vi "GDSAPI_SetClassOptions.vi"(8 "error in (no error)":errorcluster, 9 "WireConfiguration":T1={"Edge thickness"=1, "Edge color"=5667411, "Center thickness"=1, "Center pattern"=enum."Solid", "CenterColor1"=9740924, "CenterColor2"=8694662, "Tunnels and terminals colors"=131187}, 10 "PatternIn":T3 items=["4x4x4", "5x6x5", "6x8x6"], 11 "ProjectIconType":T4=enum."BlueFull") -> (0 "error out":errorcluster, 1 "WireConfiguration-Before":T1={"Edge thickness"=1, "Edge color"=5667411, "Center thickness"=1, "Center pattern"=enum."Solid", "CenterColor1"=9740924, "CenterColor2"=8694662, "Tunnels and terminals colors"=131187}, 2 "Pattern-Before":T3 items=["4x4x4", "5x6x5", "6x8x6"], 3 "ProjectIcon-Before":T4=enum."BlueFull")   [LabVIEW 2012]
uses:
  <resource>/Framework/Providers/Open_GDS/API/GDSAPI_SubVIs/GDSAPI_ProjectIconType.ctl
  <resource>/Framework/Providers/Open_GDS/ClassProviders/Common/ScriptingFunctions/Scripting_ConnectorPanePatternType.ctl
  <resource>/Framework/Providers/Open_GDS/SubVIs/GOOP_WireConfigurationType.ctl
  <resource>/Framework/Providers/Open_GDS/SubVIs/GOOP_WirePattern.ctl
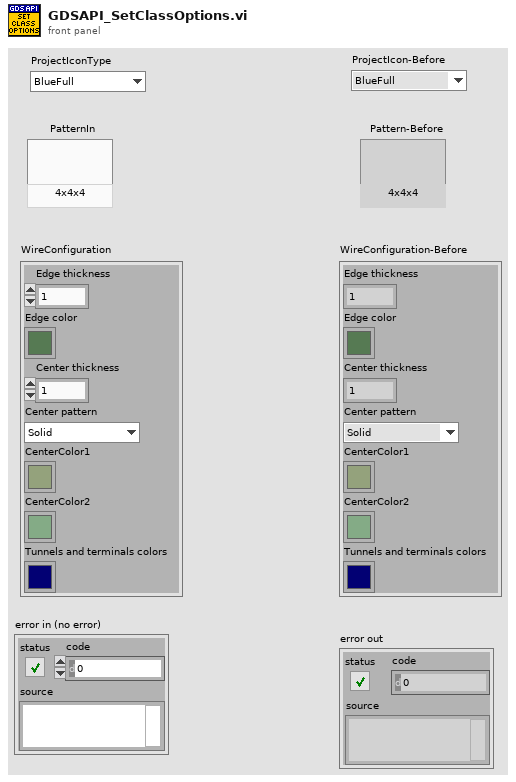
[diagram p1: front panel]
types:
  T1 = typedef "GOOP_WireConfigurationType.ctl" = cluster{"Edge thickness":i32, "Edge color":u32, "Center thickness":i32, "Center pattern":T2, "CenterColor1":u32, "CenterColor2":u32, "Tunnels and terminals colors":u32}
  T2 = typedef "GOOP_WirePattern.ctl" = enum16{"Solid", "Large dash", "Small dash"}
  T3 = typedef "Scripting_ConnectorPanePatternType.ctl" = u16
  T4 = typedef "GDSAPI_ProjectIconType.ctl" = enum16{"BlueCircle", "BlueFrame", "BlueFull", "BlueMessage", "BrownCircle", "BrownFrame", "BrownFull", "BurgundyCircle", "BurgundyFrame", "BurgundyFull", "CyanCircle", "CyanFrame", "CyanFull", "DarkBlueCircle", "DarkBlueFrame", "DarkBlueFull", "ForestGreenCircle", "ForestGreenFrame", "ForestGreenFull", "GrayCircle", "GrayFrame", "GrayFull", "GreenCircle", "GreenFrame", "GreenFull", "LightGreenCircle", "LightGreenFrame", "LightGreenFull", "LightRedCircle", "LightRedFrame", "LightRedFull", "PinkCircle", "PinkFrame", "PinkFull", "PurpleCircle", "PurpleFrame", "PurpleFull", "RedCircle", "RedFrame", "RedFull", "YellowCircle", "YellowFrame", "YellowFull"}
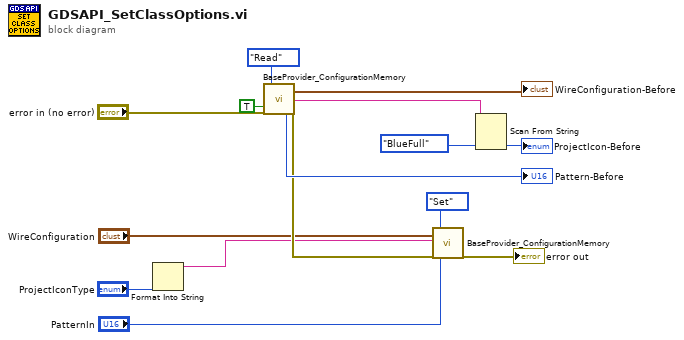
[diagram p0: block diagram]
diagram:
  n1 = Format Into String("ProjectIconType") -> (resulting string=w4:string)  [unwired: 3 in, 1 out]
  n2 = call <resource>:"BaseProvider_ConfigurationMemory.vi"("Filter_Icons"=TRUE, "error in (no error)"="error in (no error)", "Action"=enum16{"Read", "Load", "Save", "Set"}."Read") -> ("PatternOut"=→"Pattern-Before":T3, "WireConfigurationOut"=→"WireConfiguration-Before":T1, "IconOut"=w12:string, "error out"=w7:errorcluster)  [unwired: 10 in, 3 out]
  n3 = call <resource>:"BaseProvider_ConfigurationMemory.vi"("WireConfiguration"="WireConfiguration", "Icon"=w4, "error in (no error)"=w7, "Action"=enum16{"Read", "Load", "Save", "Set"}."Set", "PatternIn"="PatternIn") -> ("error out"=→"error out":errorcluster)  [unwired: 8 in, 6 out]
  n4 = Scan From String(input string=w12, default 1=GDSAPI_ProjectIconType."BlueFull" ("ProjectIcon-Before")) -> (output 1=→"ProjectIcon-Before":T4)  [unwired: 3 in, 3 out]
